vi "TimeStampIndex.vi"(11 "Analysis In":refnum<class "AnalysisPluginsBase.lvclass">) -> (1 "WEI":i32[](array[numeric]), 2 "WSI":i32[](array[numeric]), 3 "Analysis Out":refnum<class "AnalysisPluginsBase.lvclass">)   [LabVIEW 2014, in "AnalysisPlugins.lvlib" / "AnalysisPluginsBase.lvclass"]
uses:
  AnalysisPluginsBase.lvclass
  AnalysisPluginsBase.lvclass/AnalysisPluginsBase.ctl
  Accessors/Read SampleDataInput.vi
  Accessors/Read clConfig.vi
  Accessors/Read AnalysisTime.vi
panel:
  # "Window\nStart Index"
  # "Window\nEnd Index"
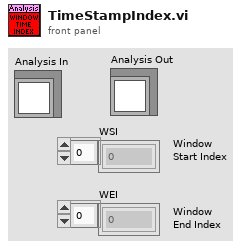
[diagram p1: front panel]
types:
  T1 = typedef "AnalysisPlugins.lvlib/AnalysisPluginsBase.lvclass/SampleDataInput.ctl" = waveform(dbl)[]
  T2 = typedef "AnalysisPlugins.lvlib/AnalysisPluginsBase.lvclass/clConfig.ctl" = cluster{"F0":u32, "SettlingTime":dbl, "AnalysisCycles":dbl, "SampleRate":dbl, "NumChannels":u32, "TsOffset":enum16{"start", "middle", "end"}}
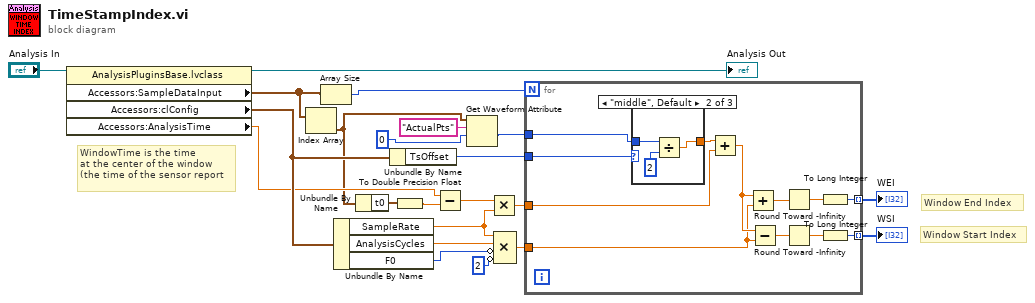
[diagram p0: block diagram]
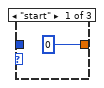
[diagram p2: hidden frame]
diagram:
  # "WindowTime is the time\nat the center of the window\n(the time of the sensor report"
  # "Window End Index"
  # "Window Start Index"
  n1 = property class="AnalysisPluginsBase.lvclass"(reference="Analysis In") -> (reference out=→"Analysis Out":refnum<class "AnalysisPluginsBase.lvclass">, "Accessors:SampleDataInput"=w2:T1, "Accessors:clConfig"=w18:T2, "Accessors:AnalysisTime"=w17:dbl)  [unwired: 1 in, 1 out]
  n2 = Index Array(array=w2) -> (element=w6:waveform(dbl))  [unwired: 1 in]
  n3 = Array Size(array=w2) -> (size(s)=w1:i32)
  n4 = Unbundle By Name(w18) -> ("SampleRate"=w14:dbl, "AnalysisCycles"=w13:dbl, "F0"=w12:u32)
  n5 = Unbundle By Name(w6) -> ("t0"=w8:timestamp)
  n6 = Unbundle By Name(w18) -> ("TsOffset"=w20:enum16{"start", "middle", "end"})
  n7 = To Double Precision Float(number=w8) -> (double precision float=w7:dbl)
  n8 = Subtract(x=w17, y=w7) -> (x-y=w16:dbl)
  n9 = Get Waveform Attribute(5:u32 0, 6:"ActualPts" ("name"), 7:w6) -> (1:w3:u32)  [unwired: 1 in, 3 out]
  n10 = Multiply(x=w16, y=w14) -> (x*y=w15:dbl)
  n11 = Compound Arithmetic op=MULTIPLY(w14, w13, invert w12, invert u32 2 ("value")) -> (w10:dbl)
  n12 = for {
    N: w1 -> [_]
    tunnel: w20 -> [w32]
    tunnel: [w29] -> w19 mode=indexing
    tunnel: w15 -> [w30]
    tunnel: w10 -> [w27]
    tunnel: [w25] -> w9 mode=indexing
    tunnel: w3 -> [w23]
    n13 = case shown="\"middle\", Default" w32 {
      tunnel: w23 -> [_ w36 w37]
      tunnel: [0 w34 w37] -> w31
      frame "start" {
      }
      frame "middle", Default {
        n14 = Divide(x=w36, y=2) -> (x/y=w34:dbl)
      }
      frame "end" {
      }
    }
    n15 = Add(x=w31, y=w30) -> (x+y=w28:dbl)
    n16 = Add(x=w28, y=w27) -> (x+y=w26:dbl)
    n17 = Subtract(x=w28, y=w27) -> (x-y=w24:dbl)
    n18 = Round Toward -Infinity(1:w26) -> ()  [unwired: 1 out]
    n19 = Round Toward -Infinity(1:w24) -> ()  [unwired: 1 out]
    n20 = To Long Integer(number=w26) -> (32bit integer=w29:i32)
    n21 = To Long Integer(number=w24) -> (32bit integer=w25:i32)
  }
  "WEI" <- w19
  "WSI" <- w9
